vi "FTW-Benchmark-MessageTransports.vi"() -> ()   [LabVIEW 2013]
uses:
  src/core/actor/endpoint/FTW-Endpoint-Type.ctl
  src/core/actor/endpoint/FTW-Actor-Endpoint.lvclass
  src/core/actor/request/FTW-Request.lvclass
  src/core/actor/router/FTW-Router.lvclass
panel:
  out "Message":string
  in  "Client Mode":enum32{"Parallel", "Serial"}(radio)=enum."Serial"
  in  "Number of Clients":i32=2
  out "Results":T1(array[cluster])
  in  "Server Addresses to Test":string[](array[string])=["tcp://127.0.0.1:*", "inproc://RandomAddress-*", "ipc://RandomIPCAddress-*"]
  in  "Requests to Send":i32=2
  in  "stop":bool
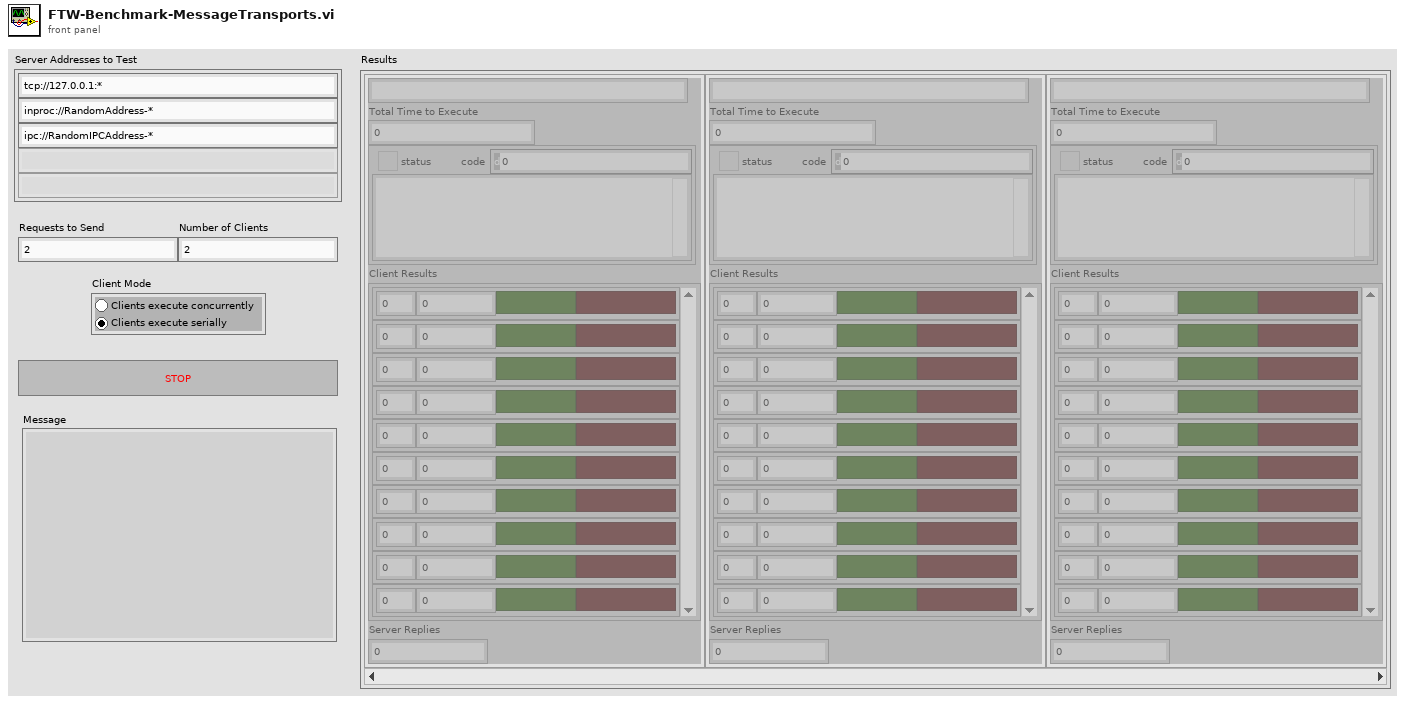
[diagram p1: front panel]
types:
  T1 = cluster{"Server Address":string, "Total Time to Execute":u32, "error":errorcluster, "Client Results":cluster{"Instance":i32, "Requests":i32, "All replies were as expected?":bool, "Timed out?":bool}[], "Server Replies":i32}[]
  T2 = typedef "FTW-Actor-Endpoint.lvclass/FTW-Endpoint-Type.ctl" = enum32{"Server", "Client", "Publisher", "Subscriber", "Pipeline Producer", "Pipeline Consumer", "Surveyor", "Respondent", "Exclusive Pair", "Bus"}
  T3 = cluster{"Actual Endpoint Address":string, "Elapsed Time":u32, "error out":errorcluster, cluster{i32, i32, bool, bool}[], i32}[]
  T4 = cluster{"Inbox Address":string, "Elapsed Time":u32, "error IO":errorcluster, cluster{i32, i32, bool, bool}[], i32}
  T5 = cluster{"Inbox Address":string, "Elapsed Time":u32, "error IO":errorcluster, cluster{i32, i32, bool, bool}[], i32}[]
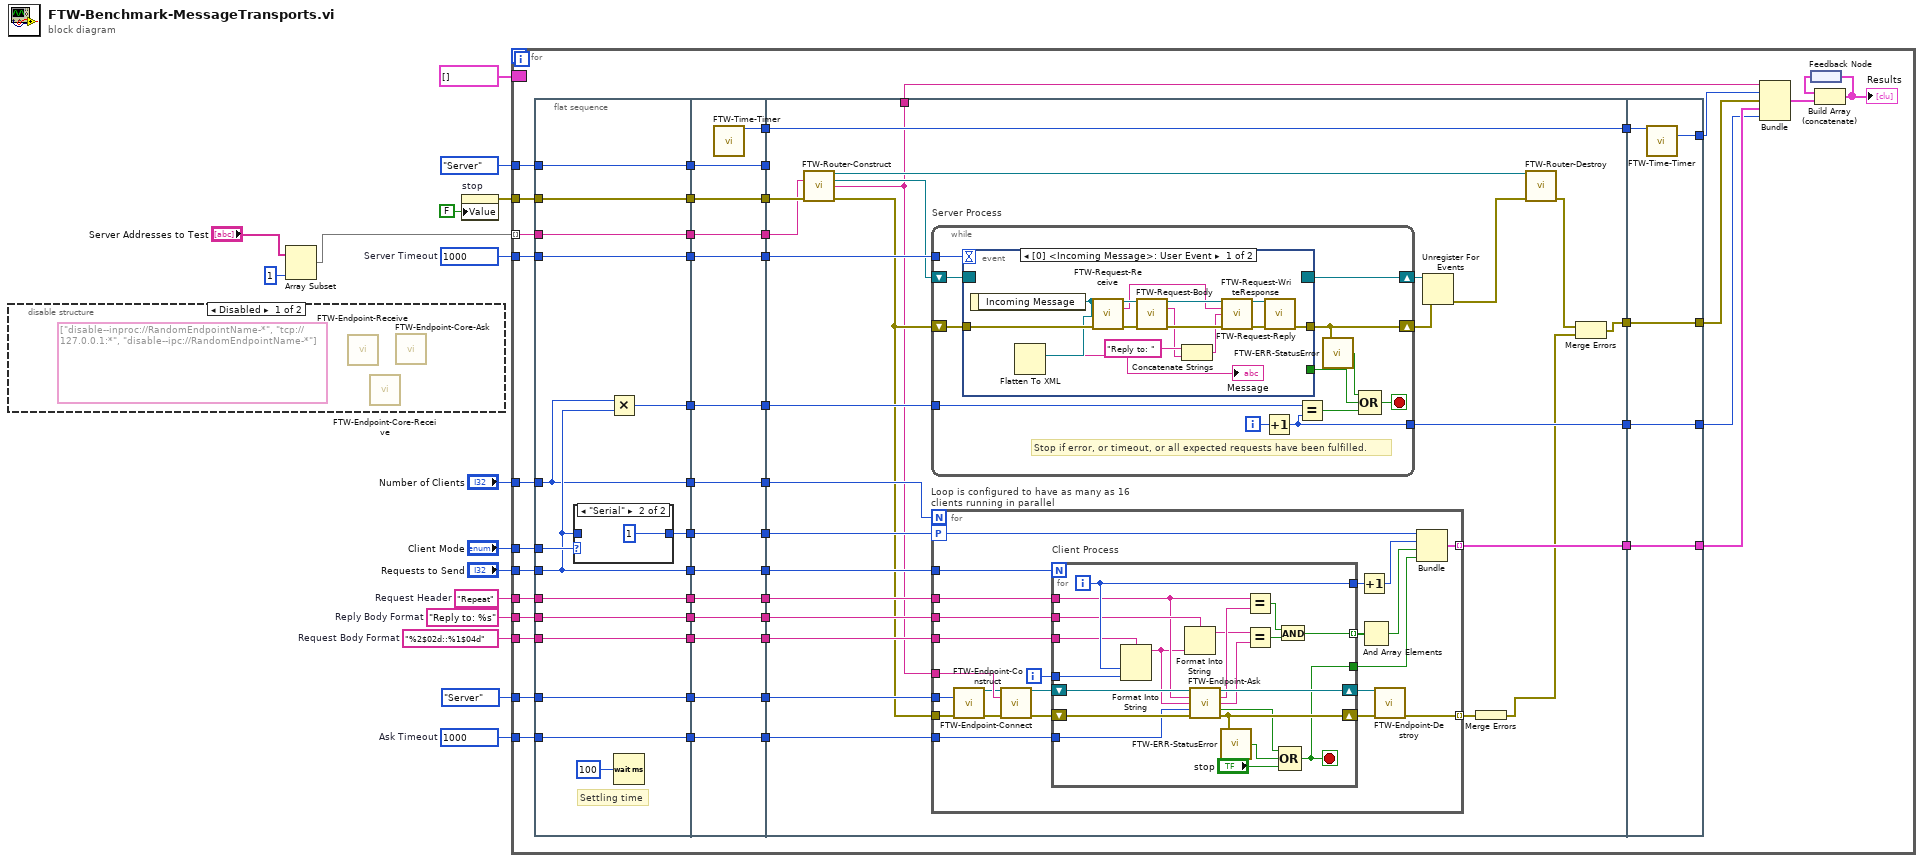
[diagram p0: block diagram]
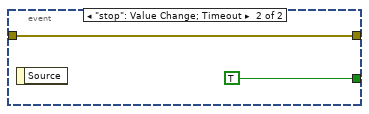
[diagram p4: hidden frame]
diagram:
  w6 = "%2$02d::%1$04d"  # Request Body Format
  w8 = "Repeat"  # Request Header
  w7 = "Reply to: %s"  # Reply Body Format
  w10 = 1000  # Ask Timeout
  w11 = 1000  # Server Timeout
  n1 = disable-structure shown="Disabled" {
    frame Disabled {
      (unwired) string[] ["disable--inproc://RandomEndpointName-*", "tcp://127.0.0.1:*", "disable--ipc://RandomEndpointName-*"] ("Server Addresses to Test")
      n2 = call-dynamic "FTW-Endpoint-Receive.vi"() -> ()  [unwired: 11 in, 5 out]
      n3 = call "FTW-Endpoint-Core-Receive.vi"() -> ()  [unwired: 10 in, 6 out]
      n4 = call "FTW-Endpoint-Core-Ask.vi"() -> ()  [unwired: 11 in, 5 out]
    }
    frame Enabled {
    }
  }
  n5 = Array Subset(array="Server Addresses to Test", length=1) -> (w2:string[])  [unwired: 1 in]
  n6 = property on="stop" class="Bool (strict)"("Value"=FALSE ("stop")) -> (error out=w12:errorcluster)  [unwired: 2 in, 1 out]
  n7 = for {
    tunnel: w2 -> [w60] mode=indexing
    tunnel: "Number of Clients" -> [w56]
    tunnel: "Requests to Send" -> [w49]
    tunnel: "Client Mode" -> [w47]
    tunnel: w12 -> [w46]
    tunnel: w11 -> [w43]
    tunnel: w10 -> [w40]
    border: T3 [] -> [_]
    tunnel: w8 -> [w30]
    tunnel: w7 -> [w27]
    tunnel: w6 -> [w24]
    tunnel: FTW-Endpoint-Type."Server" -> [w20]
    tunnel: FTW-Endpoint-Type."Server" -> [w19]
    n8 = flat-sequence {
      tunnel: [w82] -> w67
      tunnel: [w80] -> w61
      tunnel: [w71] -> w57
      tunnel: [w75] -> w50
      tunnel: w46 -> [w82]
      tunnel: w47 -> [w77]
      tunnel: w49 -> [w75]
      tunnel: w56 -> [w71]
      tunnel: w60 -> [w80]
      tunnel: [w79] -> w44
      tunnel: w43 -> [w79]
      tunnel: [w78] -> w41
      tunnel: w40 -> [w78]
      tunnel: [w76] -> w38
      tunnel: [w68] -> w36
      tunnel: [w74] -> w31
      tunnel: w30 -> [w74]
      tunnel: [w73] -> w28
      tunnel: w27 -> [w73]
      tunnel: [w72] -> w25
      tunnel: w24 -> [w72]
      tunnel: [w70] -> w21
      tunnel: w20 -> [w70]
      tunnel: w19 -> [w69]
      tunnel: [w69] -> w18
      tunnel: [w98] -> w66
      tunnel: [w97] -> w65
      tunnel: w67 -> [w98]
      tunnel: [w96] -> w62
      tunnel: w61 -> [w96]
      tunnel: [w95] -> w58
      tunnel: w57 -> [w95]
      tunnel: [w94] -> w51
      tunnel: w50 -> [w94]
      tunnel: [w93] -> w45
      tunnel: w44 -> [w93]
      tunnel: [w92] -> w42
      tunnel: w41 -> [w92]
      tunnel: [w91] -> w39
      tunnel: w38 -> [w91]
      tunnel: [w90] -> w37
      tunnel: w36 -> [w90]
      tunnel: [w89] -> w32
      tunnel: w31 -> [w89]
      tunnel: [w88] -> w29
      tunnel: w28 -> [w88]
      tunnel: [w87] -> w26
      tunnel: w25 -> [w87]
      tunnel: [w86] -> w22
      tunnel: w21 -> [w86]
      tunnel: w18 -> [w85]
      tunnel: [w85] -> w17
      tunnel: [w108] -> w64
      tunnel: [w124] -> w63
      tunnel: [w123] -> w54
      tunnel: [w109] -> w53
      tunnel: w37 -> [w120]
      tunnel: w39 -> [w115]
      tunnel: w66 -> [w111]
      tunnel: w65 -> [w124]
      tunnel: w62 -> [w103]
      tunnel: w58 -> [w118]
      tunnel: w51 -> [w119]
      tunnel: [w99] -> w48
      tunnel: w45 -> [w117]
      tunnel: w42 -> [w116]
      tunnel: w32 -> [w114]
      tunnel: w29 -> [w113]
      tunnel: w26 -> [w112]
      tunnel: w22 -> [_]
      tunnel: w17 -> [w110]
      tunnel: [w201] -> w23
      tunnel: w64 -> [w201]
      tunnel: w63 -> [w200]
      tunnel: [w199] -> w59
      tunnel: [w198] -> w55
      tunnel: w54 -> [w198]
      tunnel: [w197] -> w52
      tunnel: w53 -> [w197]
      frame #0 {
        # "Settling time"
        n9 = case shown="\"Serial\"" w77 {
          tunnel: w75 -> [w83 _]
          tunnel: [w83 1 ("Requests to Send")] -> w76
          frame "Parallel" {
          }
          frame "Serial" {
          }
        }
        n10 = Multiply(x=w71, y=w75) -> (x*y=w68:i32)
        n11 = Wait (ms)(milliseconds to wait=u32 100) -> ()  [unwired: 1 out]
      }
      frame #1 {
        n12 = call "FTW-Time-Timer.vi"() -> ("Current Tick Count"=w97:u32)  [unwired: 13 in, 2 out]
      }
      frame #2 {
        n13 = call "FTW-Router-Construct.vi"("Incoming Message Router Address"=w103, "error in"=w111) -> ("FTW Router"=w102:refnum<class "FTW-Router.lvclass">, "Incoming Request"=w101:refnum<event-registration>, "Inbox Address"=w99:string, "error out"=w100:errorcluster)  [unwired: 10 in]
        n14 = while "Server Process" {
          shift-right: [w179] -> w121
          shift-left: w101 -> [w180]
          shift-right: [w177] -> w122
          shift-left: w100 -> [w178]
          tunnel: w120 -> [w172]
          tunnel: [w169] -> w109
          tunnel: w117 -> [w171]
          i -> [w170]
          stop <- w173 stop-if-true
          # "Stop if error, or timeout, or all expected requests have been fulfilled."
          n15 = event shown="[0] <Incoming Message>: User Event" {
            selector: w180 -> [_ _]
            dyn-events: [_ _] -> w179
            timeout: w171 -> [_ _]
            tunnel: [_ TRUE] -> w175
            tunnel: w178 -> [w193 w195]
            tunnel: [w194 w195] -> w177
            event User Event {
              n16 = event-data() -> ("Incoming Message"=w182:refnum<class "FTW-Request.lvclass">)  [unwired: 1 in]
              n17 = Flatten To XML(anything=w182) -> (xml string=→"Message":string)
              n18 = call "FTW-Request-Receive.vi"("Uninitialized Request"=w182, "error in"=w193) -> ("Initialized Request"=w192:refnum<class "FTW-Request.lvclass">, "Request Header"=w185:string, "error out"=w191:errorcluster)  [unwired: 11 in]
              n19 = call "FTW-Request-Body.vi"("FTW Request"=w192, "error in"=w191) -> ("FTW Request out"=w190:refnum<class "FTW-Request.lvclass">, "Request Body"=w184:string, "error out"=w187:errorcluster)  [unwired: 11 in]
              n20 = Concatenate Strings("Reply to: ", w184) -> (w183:string)
              n21 = call "FTW-Request-WriteResponse.vi"("FTW Incoming Request"=w190, "Response Header"=w185, "Response Body"=w183, "error in"=w187) -> ("FTW Incoming Request out"=w189:refnum<class "FTW-Request.lvclass">, "error out"=w188:errorcluster)  [unwired: 10 in]
              n22 = call "FTW-Request-Reply.vi"("FTW Incoming Request"=w189, "error in"=w188) -> ("error out"=w194:errorcluster)  [unwired: 12 in, 1 out]
            }
            event "stop": Value Change; Timeout {
              n23 = event-data() -> ()  [unwired: 1 in, 1 out]
            }
          }
          n24 = Increment(x=w170) -> (x+1=w169:i32)
          n25 = Equal?(x=w172, y=w169) -> (x = y?=w174:bool)
          n26 = call "FTW-ERR-StatusError.vi"("error to check"=w177) -> ("Error?"=w176:bool)
          n27 = Compound Arithmetic op=OR(w176, w175, w174) -> (w173:bool)
        }
        n28 = for "Loop is configured to have as many as 16 clients running in parallel" {
          N: w118 -> [_]
          tunnel: w100 -> [w132]
          tunnel: w119 -> [w147]
          tunnel: w116 -> [w146]
          workers-P: w115 -> [w142]
          tunnel: [w145] -> w123 mode=indexing
          tunnel: w99 -> [w134]
          tunnel: w113 -> [w140]
          tunnel: w114 -> [w139]
          tunnel: w112 -> [w138]
          tunnel: w110 -> [w130]
          tunnel: [w126] -> w107 mode=indexing
          i -> [w129]
          n29 = call "FTW-Endpoint-Construct.vi"("Endpoint Type"=w130, "error in"=w132) -> ("FTW Endpoint"=w133:refnum<class "FTW-Actor-Endpoint.lvclass">, "error out"=w131:errorcluster)  [unwired: 12 in]
          n30 = call "FTW-Endpoint-Connect.vi"("FTW Socket"=w133, "Remote Address"=w134, "error in"=w131) -> ("FTW Socket out"=w136:refnum<class "FTW-Actor-Endpoint.lvclass">, "error out"=w135:errorcluster)  [unwired: 11 in]
          n31 = for "Client Process" {
            N: w147 -> [_]
            shift-right: [w166] -> w128
            shift-left: w136 -> [w168]
            tunnel: w146 -> [w162]
            tunnel: [w148] -> w143
            tunnel: [w160] -> w144
            tunnel: [w151] -> w125 mode=indexing
            tunnel: w140 -> [w159]
            tunnel: w139 -> [w155]
            tunnel: w138 -> [w158]
            shift-right: [w165] -> w127
            shift-left: w135 -> [w167]
            tunnel: w129 -> [w154]
            i -> [w160]
            stop <- w148 stop-if-true
            n32 = Format Into String(format string=w158, w160, w154) -> (resulting string=w152:string)  [unwired: 2 in, 1 out]
            n33 = Format Into String(format string=w159, w152) -> (resulting string=w150:string)  [unwired: 2 in, 1 out]
            n34 = call-dynamic "FTW-Endpoint-Ask.vi"("FTW Socket"=w168, "Request Header"=w155, "Request Body"=w152, "Timeout"=w162, "error in"=w167) -> ("FTW Socket out"=w166:refnum<class "FTW-Actor-Endpoint.lvclass">, "Response Header"=w156:string, "Response Body"=w149:string, "Timed out?"=w161:bool, "error out"=w165:errorcluster)  [unwired: 6 in]
            n35 = call "FTW-ERR-StatusError.vi"("error to check"=w165) -> ("Error?"=w164:bool)
            n36 = Equal?(x=w155, y=w156) -> (x = y?=w153:bool)
            n37 = Equal?(x=w150, y=w149) -> (x = y?=w157:bool)
            n38 = And(x=w153, y=w157) -> (x .and. y?=w151:bool)
            n39 = Compound Arithmetic op=OR(w161, w164, "stop") -> (w148:bool)
          }
          n40 = Increment(x=w144) -> (x+1=w141:i32)
          n41 = And Array Elements(Boolean array=w125) -> (logical AND=w137:bool)
          n42 = call-dynamic "FTW-Endpoint-Destroy.vi"("FTW Socket"=w128, "error in"=w127) -> ("error out"=w126:errorcluster)  [unwired: 13 in]
          n43 = Bundle(w142, w141, w137, w143) -> (w145:cluster{i32, i32, bool, bool})  [unwired: 1 in]
        }
        n44 = Unregister For Events(event registration refnum=w121, error in=w122) -> (error out=w104:errorcluster)
        n45 = Merge Errors(w107) -> (w105:errorcluster)
        n46 = call "FTW-Router-Destroy.vi"("FTW Router"=w102, "error in"=w104) -> ("error out"=w106:errorcluster)  [unwired: 13 in]
        n47 = Merge Errors(w106, w105) -> (w108:errorcluster)
      }
      frame #3 {
        n48 = call "FTW-Time-Timer.vi"("Initial Tick Count"=w200) -> ("Elapsed Time"=w199:u32)  [unwired: 12 in, 2 out]
      }
    }
    n49 = Bundle("Inbox Address"=w48, "Elapsed Time"=w59, "error IO"=w23, w55, w52) -> (w35:T4)  [unwired: 1 in]
    n50 = feedback #1() -> (w34:T3)
    n51 = Build Array (concatenate)(w34, w35) -> (w33:T5)
    "Results" <- w33
    n52 = feedback-in #1(w33) -> ()
  }
